vi "Tektronix_Measure.vi"(0 "Channel":i32(ring) items=["Channel 1", "Channel 2", "Channel 3", "Channel 4"], 5 "TestIndex":i32, 7 "Measurement":i32(ring)=1 items=["Frequency", "Mean", "Period", "Pulse Duty", "Peak to Peak", "Cycle RMS", "Minimum", "Maximum", "Rise Time", "Fall Time", "Positive Width", "Negative Width", "Amplitude", "Cycle Mean", "High", "Low", "Negative Duty", "Positive Overshoot", "Negative Overshoot", "Cursor Mean", "Burst Width", "Positive Pulse Count", "Negative Pulse Count", "Rising Edge Count", "Falling Edge Count", "Area", "Cycle Area", "RMS", "Cursor RMS"], 11 "error in":errorcluster) -> (4 "测量值":dbl, 15 "error out":errorcluster)   [LabVIEW 2015]
panel:
  out "读取缓冲区":string
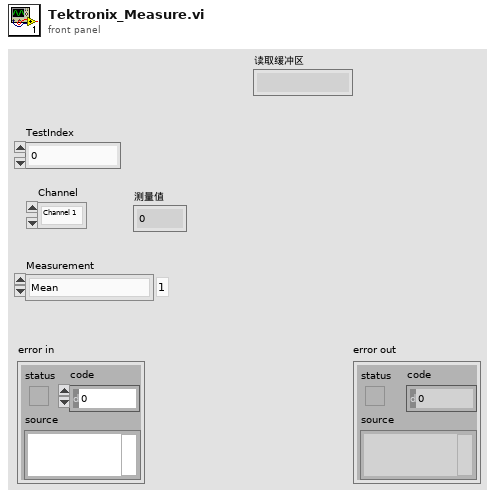
[diagram p1: front panel]
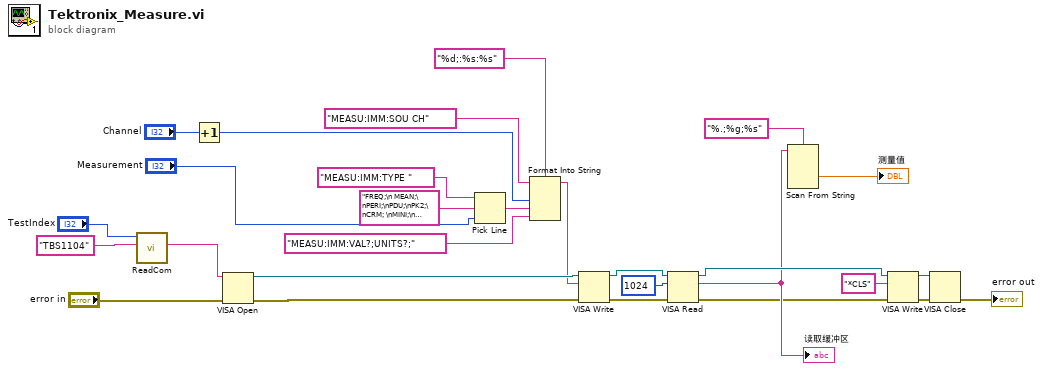
[diagram p0: block diagram]
diagram:
  n1 = call "ReadCom.vi"("仪器名称"="TBS1104", "MyIndex"="TestIndex") -> ("COM"=w18:string)  [unwired: 7 in, 2 out]
  n2 = Increment(x="Channel") -> (x+1=w3:i32)
  n3 = VISA Open(error in (no error)="error in", VISA resource name=w18) -> (VISA resource name=w26:refnum<visa-resource-name>, error out=w25:errorcluster)  [unwired: 3 in]
  n4 = Pick Line(string ("")="MEASU:IMM:TYPE ", multi-line string="FREQ;\n MEAN;\nPERI;\nPDU;\nPK2;\nCRM; \nMINI;\n MAXI;\n RIS;\nFALL;\nPWI;\nNWI;\nAMP;\nCMEAN;\nHIG;\nLOW;\nNDU;\nPOVER;\nNOVER;\nCURSORM;\nBURSTWID;\nPPULSEC;\nNPULSEC;\nREDGEC;\nFEDGEC;\nAREA;\nCAREA;\nRMS;\nCURSORR;", line index="Measurement") -> (output string=w9:string)
  n5 = Format Into String(format string="%d;:%s:%s", initial string="MEASU:IMM:SOU CH" ("string (\"\")"), w3, w9, "MEASU:IMM:VAL?;UNITS?;" ("write buffer")) -> (resulting string=w11:string)  [unwired: 1 in, 1 out]
  n6 = VISA Write(VISA resource name=w26, write buffer=w11, error in (no error)=w25) -> (VISA resource name out=w17:refnum<visa-resource-name>, error out=w16:errorcluster)  [unwired: 1 out]
  n7 = VISA Read(VISA resource name=w17, byte count=u32 1024, error in (no error)=w16) -> (VISA resource name out=w28:refnum<visa-resource-name>, read buffer=w8:string, error out=w1:errorcluster)  [unwired: 1 out]
  "读取缓冲区" <- w8
  n8 = Scan From String(format string="%.;%g;%s", input string=w8) -> (output 1=→"测量值":dbl)  [unwired: 2 in, 6 out]
  n9 = VISA Write(VISA resource name=w28, write buffer="*CLS" ("写入缓冲区"), error in (no error)=w1) -> (VISA resource name out=w22:refnum<visa-resource-name>, error out=w21:errorcluster)  [unwired: 1 out]
  n10 = VISA Close(VISA resource name=w22, error in (no error)=w21) -> (error out=→"error out":errorcluster)
